vi "Add Timestamp to File Name.vi"(1 "base path":path) -> (0 "timestamped path":path)   [LabVIEW 2021, in "Logging.lvlib"]
doc: "Add a timestamp to the name part of 'base path' and return it in 'timestamped path'. This VI preserves file extension."
uses:
  Logging.lvlib
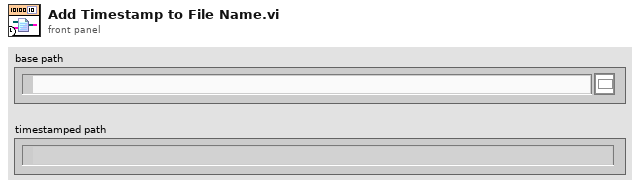
[diagram p1: front panel]
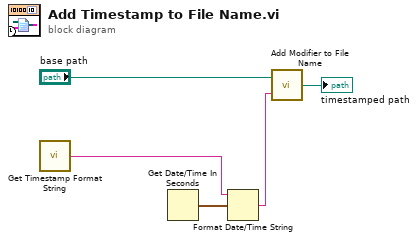
[diagram p0: block diagram]
diagram:
  n1 = call "Get Timestamp Format String.vi"() -> ("time format string"=w2:string)
  n2 = Get Date/Time In Seconds() -> (seconds since 1Jan1904=w3:timestamp)
  n3 = Format Date/Time String(time format string (%c)=w2, seconds (now)=w3) -> (date/time string=w1:string)  [unwired: 1 in]
  n4 = call "Add Modifier to File Name.vi"("file name modifier"=w1, "base path"="base path") -> ("appended path"=→"timestamped path":path)
